vi "beta.vi"(10 "time":dbl[](array[numeric]), 11 "g(k) in":dbl[][](array[numeric])) -> (2 "beta 2":dbl)   [LabVIEW 2015]
uses:
  <vilib>/Analysis/NI_AALPro.lvlib
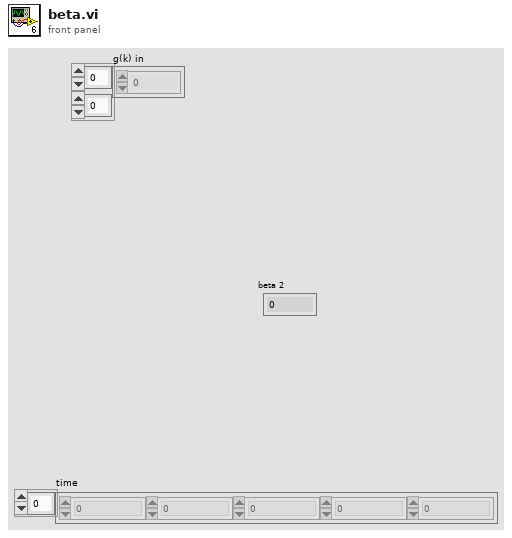
[diagram p1: front panel]
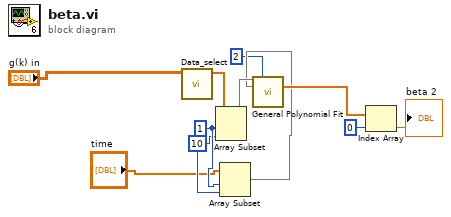
[diagram p0: block diagram]
diagram:
  w8 = 10 ("length")
  w9 = 1 ("index")
  n1 = call "Data_select.vi"("g(k) in"="g(k) in") -> ("g(k) lineal"=w5:ext[])  [unwired: 9 in, 1 out]
  n2 = Array Subset(array=w5, index=w9, length=w8) -> (w10:ext[])
  n3 = Array Subset(array="time", index=w9, length=w8) -> (w2:dbl[])
  n4 = call <vilib>:"General Polynomial Fit.vi"("Y"=w10, "polynomial order"=2, "X"=w2) -> ("Polynomial Coefficients"=w7:dbl[])  [unwired: 9 in, 3 out]
  n5 = Index Array(array=w7, index=0) -> (element=→"beta 2":dbl)
